vi "Acceleration Limiter.vi"() -> ()   [LabVIEW 2018]
panel:
  out "Acceleration Limited Speed Out":dbl
  in  "Raw Speed In":dbl
  in  "Max Allowed Increase of Change in Speed [0, 1] (0)":dbl
  in  "Max Allowed Decrease of Change in Speed [0, 1] (1)":dbl
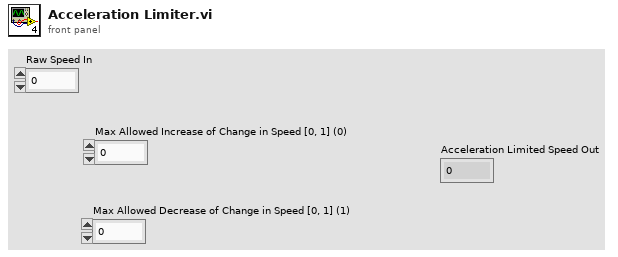
[diagram p1: front panel]
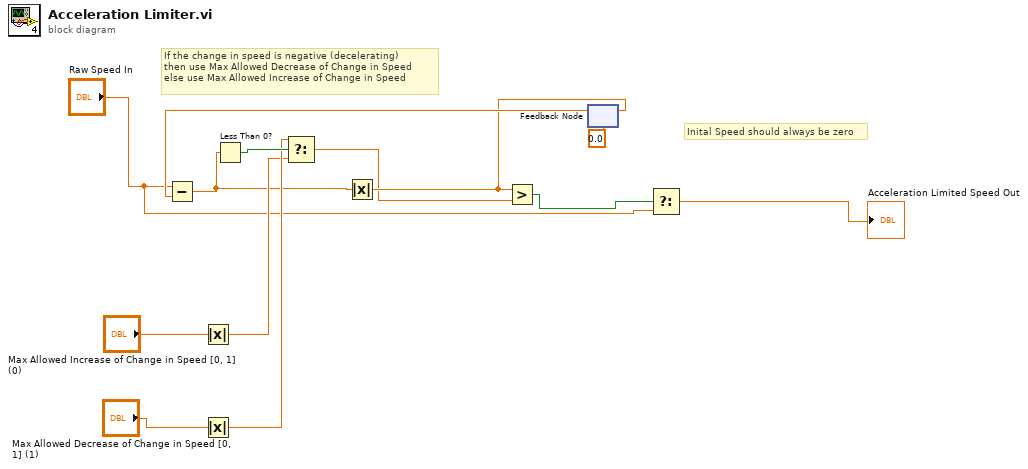
[diagram p0: block diagram]
diagram:
  # "If the change in speed is negative (decelerating)\nthen use Max Allowed Decrease of Change in Speed\nelse use Max Allowed Increase of Change in Speed"
  # "Inital Speed should always be zero"
  n1 = Absolute Value(x="Max Allowed Increase of Change in Speed [0, 1] (0)") -> (abs(x)=w6:dbl)
  n2 = Absolute Value(x="Max Allowed Decrease of Change in Speed [0, 1] (1)") -> (abs(x)=w7:dbl)
  n3 = feedback #1(0.0) -> (w12:dbl)
  n4 = Subtract(x="Raw Speed In", y=w12) -> (x-y=w5:dbl)
  n5 = Less Than 0?(x=w5) -> (x < 0?=w9:bool)
  n6 = Select(t=w7, s=w9, f=w6) -> (s? t:f=w3:dbl)
  n7 = Absolute Value(x=w5) -> (abs(x)=w4:dbl)
  n8 = Greater?(x=w4, y=w3) -> (0:w10:bool)
  n9 = feedback-in #1(w4) -> ()
  n10 = Select(s=w10, f="Raw Speed In") -> (s? t:f=→"Acceleration Limited Speed Out":dbl)  [unwired: 1 in]
